vi "_Extract XML Element.vi"(4 "error in":errorcluster, 6 "XML Type":T1, 7 "XML String":string) -> (0 "error out":errorcluster, 1 "Element":string, 2 "Attributes":string, 3 "Remaining String":string)   [LabVIEW 2015]
uses:
  Type/_XML Type.ctl
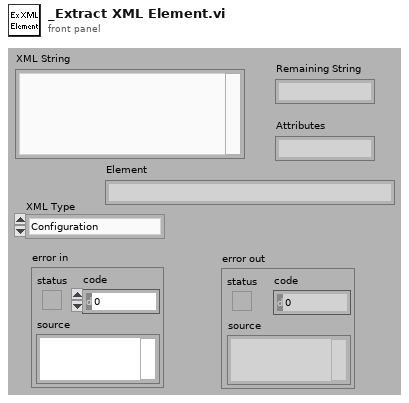
[diagram p1: front panel]
types:
  T1 = typedef "_XML Type.ctl" = enum16{"Configuration", "ConTable", "Method", "Experiment", "Mass Range", "Table", "LensTable", "ParamTable", "TuneParam", "MetParam", "MassRange", "LCMethod", "LCMethodFile", "RackType", "Vial", "PlatePos", "InjVol"}
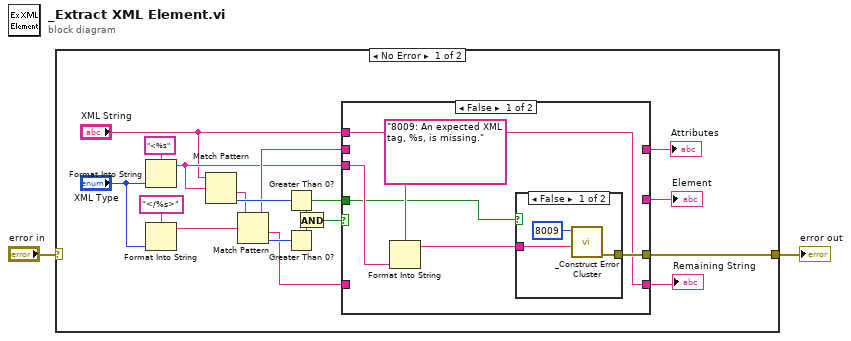
[diagram p0: block diagram]
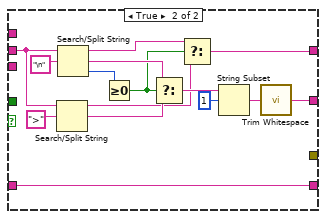
[diagram p3: hidden frame]
diagram:
  n1 = case shown="No Error" "error in" {
    selector: "error in" -> [_ w45]
    tunnel: [w19 w45] -> w1
    frame No Error {
      n2 = Format Into String(format string="<%s", "XML Type") -> (resulting string=w11:string)  [unwired: 2 in, 1 out]
      n3 = Format Into String(format string="</%s>", "XML Type") -> (resulting string=w9:string)  [unwired: 2 in, 1 out]
      n4 = Match Pattern(string="XML String", regular expression=w11) -> (after substring=w18:string, offset past match=w20:i32)  [unwired: 3 out]
      n5 = Match Pattern(string=w18, regular expression=w9) -> (before substring=w14:string, after substring=w10:string, offset past match=w17:i32)  [unwired: 2 out]
      n6 = Greater Than 0?(x=w20) -> (x > 0?=w3:bool)
      n7 = Greater Than 0?(x=w17) -> (x > 0?=w16:bool)
      n8 = And(x=w3, y=w16) -> (x .and. y?=w15:bool)
      n9 = case shown="False" w15 {
        tunnel: w14 -> [_ w39]
        tunnel: [w26 _] -> w19
        tunnel: "XML String" -> [w22 _]
        tunnel: w11 -> [w25 _]
        tunnel: w10 -> [_ w44]
        tunnel: [w22 w44] -> w8
        tunnel: [_ w30] -> w7
        tunnel: [_ w42] -> w6
        tunnel: w3 -> [w21 _]
        frame False {
          n10 = Format Into String(format string="8009: An expected XML tag, %s, is missing.", w25) -> (resulting string=w23:string)  [unwired: 2 in, 1 out]
          n11 = case shown="False" w21 {
            tunnel: [w29 _] -> w26
            tunnel: w23 -> [w28 _]
            frame False {
              n12 = call "_Construct Error Cluster.vi"("reason"=w28, "errorCode"=8009) -> ("error out"=w29:errorcluster)  [unwired: 2 in, 3 out]
            }
            frame True {
            }
          }
        }
        frame True {
          n13 = Search/Split String(string=w39, search string/char (-)=">") -> (substring before match=w31:string, match + rest of string=w35:string)  [unwired: 2 out]
          n14 = Search/Split String(string=w39, search string/char (-)="\n") -> (substring before match=w33:string, match + rest of string=w36:string, offset of match=w41:i32)  [unwired: 1 out]
          n15 = Greater Or Equal To 0?(x=w41) -> (x >= 0?=w32:bool)
          n16 = Select(t=w36, s=w32, f=w35) -> (s? t:f=w34:string)
          n17 = Select(t=w33, s=w32, f=w31) -> (s? t:f=w30:string)
          n18 = String Subset(string=w34, offset (0)=1 ("default value 1")) -> (substring=w37:string)  [unwired: 1 out]
          n19 = call <vilib>:"Trim Whitespace.vi"("string"=w37) -> ("trimmed string"=w42:string)  [unwired: 1 in]
        }
      }
      "Remaining String" <- w8
      "Attributes" <- w7
      "Element" <- w6
    }
    frame Error {
    }
  }
  "error out" <- w1
